vi "TCP_read.vi"(0 "Client ID In":refnum<k5>, 1 "error in (no error)":errorcluster) -> (2 "Client ID out":refnum<k5>, 3 "Dataout":string, 4 "error out (no error)":errorcluster)   [LabVIEW 2011]
doc: "Reads client settings from the tcp connection and convert it into a output string"
panel:
  in  "timeout ms (5000)":i32=5000
  out "Expected data length":i32
  out "Received data length":i32
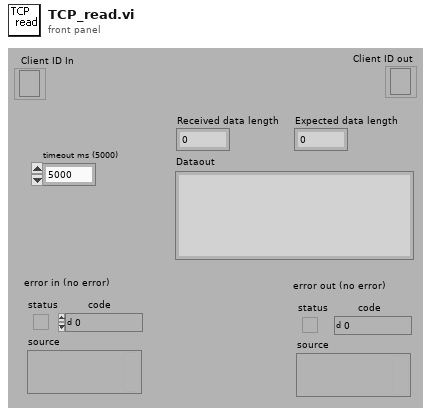
[diagram p1: front panel]
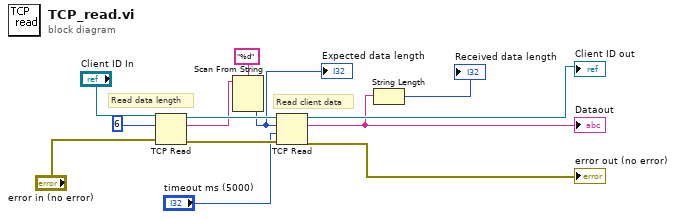
[diagram p0: block diagram]
diagram:
  # "Read data length"
  # "Read client data"
  n1 = TCP Read(connection ID="Client ID In", bytes to read=6, error in (no error)="error in (no error)") -> (connection ID out=w10:refnum<k5>, data out=w7:string, error out=w11:errorcluster)  [unwired: 2 in]
  n2 = Scan From String(format string="%d" ("Format String"), input string=w7) -> (output 1=w5:i32)  [unwired: 3 in, 3 out]
  "Expected data length" <- w5
  n3 = TCP Read(connection ID=w10, bytes to read=w5, error in (no error)=w11, 9:"timeout ms (5000)") -> (connection ID out=→"Client ID out":refnum<k5>, data out=w2:string, error out=→"error out (no error)":errorcluster)  [unwired: 1 in]
  "Dataout" <- w2
  n4 = String Length(string=w2) -> (length=→"Received data length":i32)
